vi "Set Vector Components.vi"(8 "error in":errorcluster, 9 "Y":dbl, 10 "X":dbl, 11 "PVector in":refnum<class "PVector.lvclass">) -> (0 "error out":errorcluster, 3 "PVector out":refnum<class "PVector.lvclass">)   [LabVIEW 2016, in "PVector.lvclass"]
doc: "Set vector V individual components Vx and Vy"
uses:
  PVector.lvclass
  PVector.lvclass/PVector.ctl
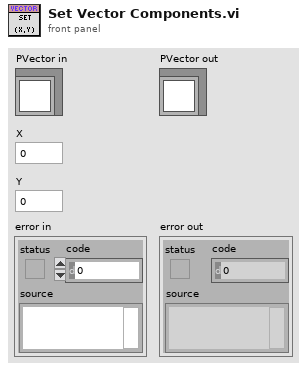
[diagram p1: front panel]
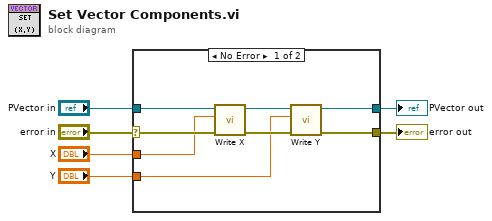
[diagram p0: block diagram]
diagram:
  n1 = case shown="No Error" "error in" {
    selector: "error in" -> [w12 w16]
    tunnel: [w10 w16] -> w5
    tunnel: [w9 w15] -> w3
    tunnel: "PVector in" -> [w14 w15]
    tunnel: "X" -> [w8 _]
    tunnel: "Y" -> [w7 _]
    frame No Error {
      n2 = call "Write X.vi"("error in"=w12, "X"=w8, "PVector in"=w14) -> ("error out"=w11:errorcluster, "PVector out"=w13:refnum<class "PVector.lvclass">)  [unwired: 7 in]
      n3 = call "Write Y.vi"("error in"=w11, "Y"=w7, "PVector in"=w13) -> ("error out"=w10:errorcluster, "PVector out"=w9:refnum<class "PVector.lvclass">)  [unwired: 7 in]
    }
    frame Error {
    }
  }
  "error out" <- w5
  "PVector out" <- w3
